vi "NI VeriStand - Find next valid Label.vi"(7 "Try requested Label only?":bool, 8 "error in (no error)":errorcluster, 9 "Start Value (1)":i32, 10 "Label":string, 11 "Item Ref in":T1 format="%.0x") -> (0 "error out":errorcluster, 2 "Label out":string, 3 "Item Ref out":T1 format="%.0x", 4 "Found":bool, 6 "Requested label not in use?":bool)   [LabVIEW 2020, in "Custom Device API.lvlib"]
doc: "Searches the custom device hierarchy for the <B>Label</B> you specify and determines whether another item is already using the label. If the label already is in use, this VI adds a value to the end of the label and increments that value until it finds a label that is not in use. Use this VI to avoid accidentally overwriting custom device items by specifying duplicate label names."
uses:
  <vilib>/NI VeriStand/Custom Device API/Custom Device API.lvlib
  <vilib>/NI VeriStand/Custom Device API/Custom Device Item Ref.ctl
  29cbbfc3-8b54-4f32-a697-b67f6c63a573.vi
  <vilib>/NI VeriStand/Custom Device API/Custom Device Offline Path.vi
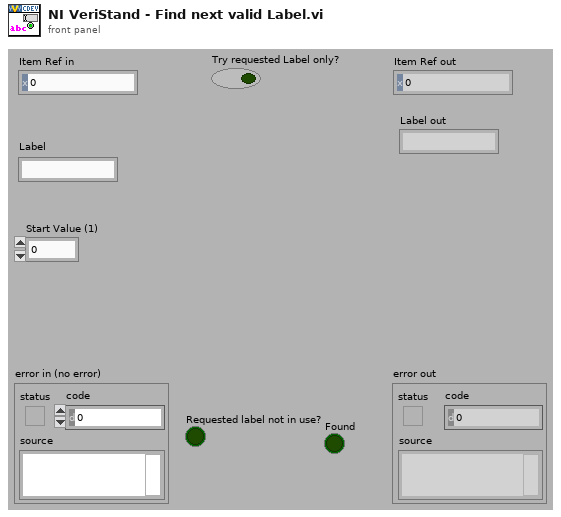
[diagram p1: front panel]
types:
  T1 = typedef "Custom Device API.lvlib/Custom Device Item Ref.ctl" = u64
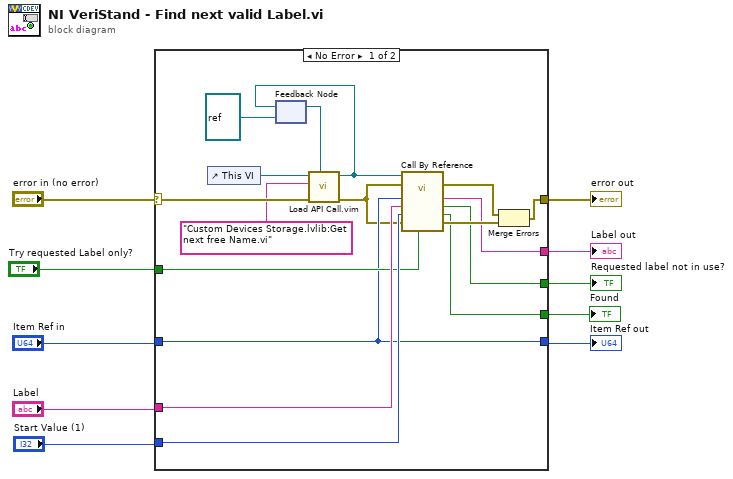
[diagram p0: block diagram]
diagram:
  n1 = case shown="No Error" "error in (no error)" {
    selector: "error in (no error)" -> [w16 w29]
    tunnel: [w26 w29] -> w10
    tunnel: "Label" -> [w25 _]
    tunnel: "Item Ref in" -> [w19 w28]
    tunnel: "Start Value (1)" -> [w24 _]
    tunnel: "Try requested Label only?" -> [w23 _]
    tunnel: [w22 _] -> w5
    tunnel: [w21 _] -> w4
    tunnel: [w20 _] -> w3
    tunnel: [w19 w28] -> w1
    frame No Error {
      n2 = control-ref of="This VI"() -> (w17:refnum<vi>)
      n3 = feedback #1(refnum<vi> refnum ("type specifier VI Refnum (for type only)")) -> (w18:refnum<vi>)
      n4 = call "Load API Call.vim"("VI reference in"=w18, "error in (no error)"=w16, "VI qualified name"="Custom Devices Storage.lvlib:Get next free Name.vi", "Caller VI ref"=w17) -> ("error out"=w14:errorcluster, "VI reference"=w15:refnum<vi>)  [unwired: 6 in]
      n5 = feedback-in #1(w15) -> ()
      n6 = call-by-ref "?"(reference=w15, error in=w14, "Try requested Label only?"=w23, 8:"error in (no error)"=w14, "Start Value"=w24, "Label"=w25, "Item Ref in"=w19) -> (error out=w11:errorcluster, 0:"error out"=w27:errorcluster, "Found"=w20:bool, "Requested label not in use"=w21:bool, "Label out"=w22:string)  [unwired: 3 in, 1 out]
      n7 = Merge Errors(w11, w27) -> (w26:errorcluster)
    }
    frame Error {
    }
  }
  "Item Ref out" <- w1
  "error out" <- w10
  "Label out" <- w5
  "Requested label not in use?" <- w4
  "Found" <- w3
